vi "Set Controls State When Running.vi"(8 "error in (no error)":errorcluster, 11 "TS UI Data in":T1) -> (0 "error out":errorcluster)   [LabVIEW 2015]
uses:
  Type defs/TS UI Data.ctl
  Type defs/Nest cluster.ctl
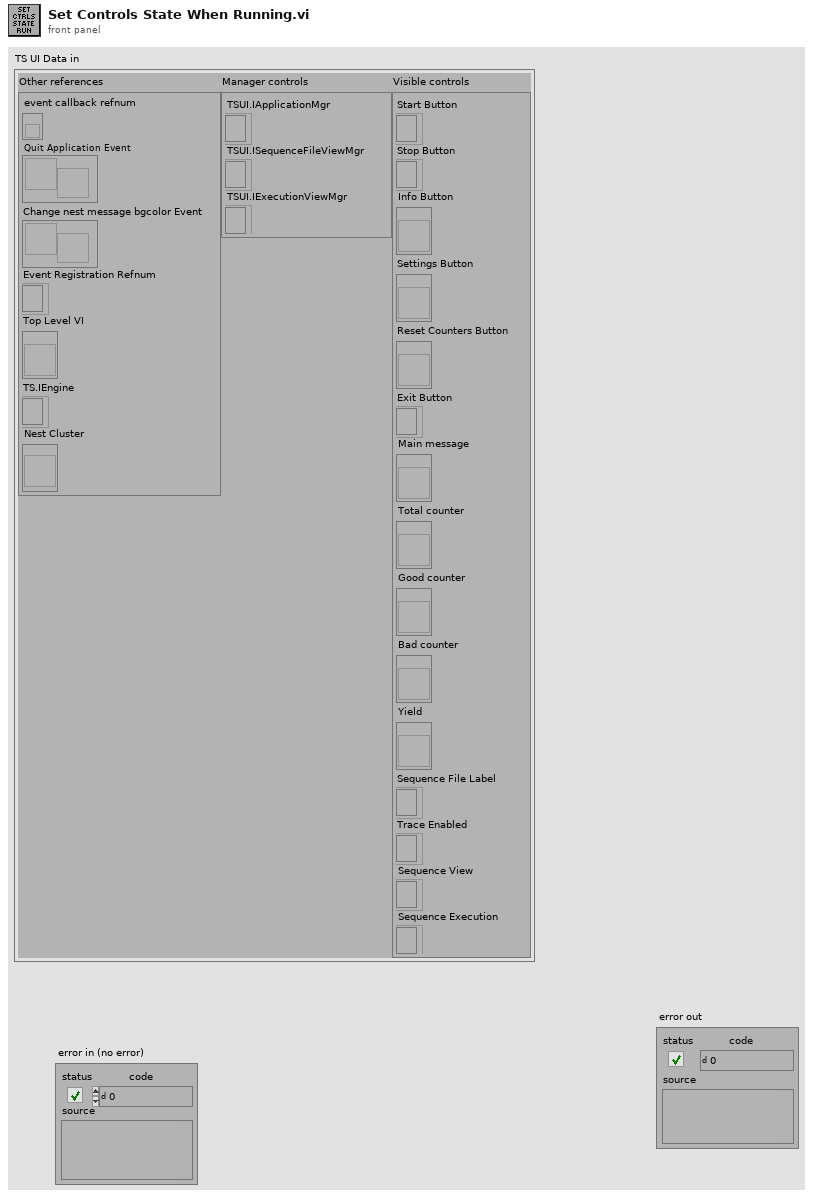
[diagram p1: front panel]
types:
  T1 = typedef "TS UI Data.ctl" = cluster{"Other references":cluster{"event callback refnum":refnum<k27>, "Quit Application Event":refnum<user-event>, "Change nest message bgcolor Event":refnum<user-event>, "event registration refnum":refnum<event-registration>, "Top Level VI":refnum<vi>, "TS.IEngine":refnum<k7>, "Nest Cluster":refnum<vi>}, "Manager controls":cluster{"TSUI.IApplicationMgr":refnum<k7>, "TSUI.ISequenceFileViewMgr":refnum<k7>, "TSUI.IExecutionViewMgr":refnum<k7>}, "Visible controls":cluster{"Start Button":refnum<k7>, "Stop Button":refnum<k7>, "Info Button":refnum<vi>, "Settings Button":refnum<vi>, "Reset Counters Button":refnum<vi>, "Exit Button":refnum<k7>, "Main message":refnum<vi>, "Total counter":refnum<vi>, "Good counter":refnum<vi>, "Bad counter":refnum<vi>, "Yield":refnum<vi>, "Sequence File Label":refnum<k7>, "Trace Enabled":refnum<k7>, "Sequence View":refnum<k7>, "Sequence Execution":refnum<k7>}}
  T2 = enum8{"Enabled", "Disabled", "Disabled and Grayed Out"}
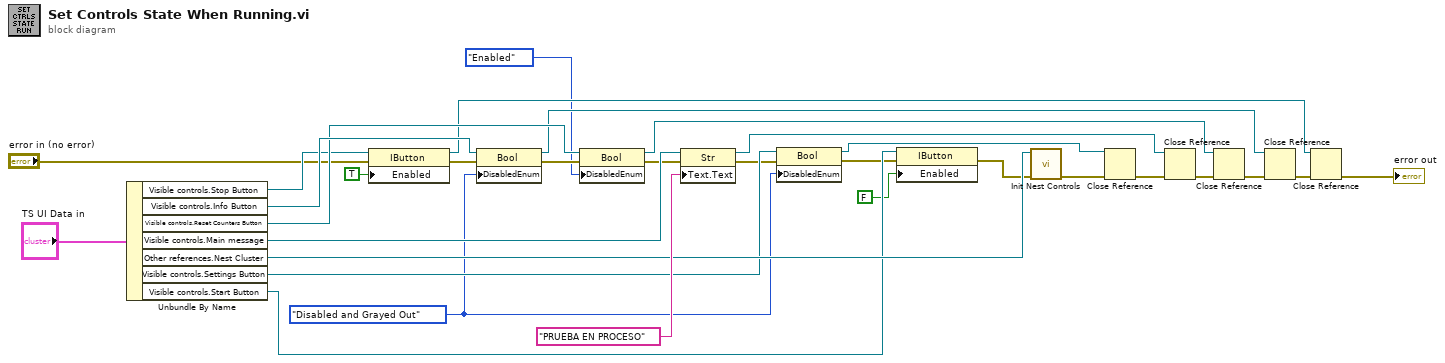
[diagram p0: block diagram]
diagram:
  w10 = T2."Disabled and Grayed Out" ("Disabled")
  n1 = Unbundle By Name("TS UI Data in") -> ("Visible controls.Stop Button"=w25:refnum<k7>, "Visible controls.Info Button"=w31:refnum<vi>, "Visible controls.Reset Counters Button"=w30:refnum<vi>, "Visible controls.Main message"=w27:refnum<vi>, "Other references.Nest Cluster"=w12:refnum<vi>, "Visible controls.Settings Button"=w11:refnum<vi>, "Visible controls.Start Button"=w5:refnum<k7>)
  n2 = property class="IButton"(reference=w25, error in="error in (no error)", "Enabled"=TRUE) -> (reference out=w15:refnum<k7>, error out=w23:errorcluster)
  n3 = property class="Bool"(reference=w31, error in=w23, "DisabledEnum"=w10) -> (reference out=w17:refnum<vi>, error out=w29:errorcluster)
  n4 = property class="Bool"(reference=w30, error in=w29, "DisabledEnum"=T2."Enabled" ("Disabled")) -> (reference out=w19:refnum<vi>, error out=w21:errorcluster)
  n5 = property class="Str"(reference=w27, error in=w21, "Text.Text"="PRUEBA EN PROCESO") -> (reference out=w13:refnum<vi>, error out=w9:errorcluster)
  n6 = property class="Bool"(reference=w11, error in=w9, "DisabledEnum"=w10) -> (reference out=w7:refnum<vi>, error out=w4:errorcluster)
  n7 = property class="IButton"(reference=w5, error in=w4, "Enabled"=FALSE) -> (error out=w3:errorcluster)  [unwired: 1 out]
  n8 = call "Init Nest Controls.vi"("error in (no error)"=w3, "Nest Cluster"=w12) -> ("error out"=w1:errorcluster)  [unwired: 9 in]
  n9 = Close Reference(reference=w7, error in (no error)=w1) -> (error out=w8:errorcluster)
  n10 = Close Reference(reference=w13, error in (no error)=w8) -> (error out=w20:errorcluster)
  n11 = Close Reference(reference=w19, error in (no error)=w20) -> (error out=w18:errorcluster)
  n12 = Close Reference(reference=w17, error in (no error)=w18) -> (error out=w16:errorcluster)
  n13 = Close Reference(reference=w15, error in (no error)=w16) -> (error out=→"error out":errorcluster)
